vi "Search by MODEL.vi"(8 "error in (no error)":errorcluster, 10 "Device Info":T1, 11 "array of devices":T2) -> (0 "error out":errorcluster, 3 "Array":T1[](array[typedef]))   [LabVIEW 2016]
uses:
  Array Device Info.ctl
  Device Info.ctl
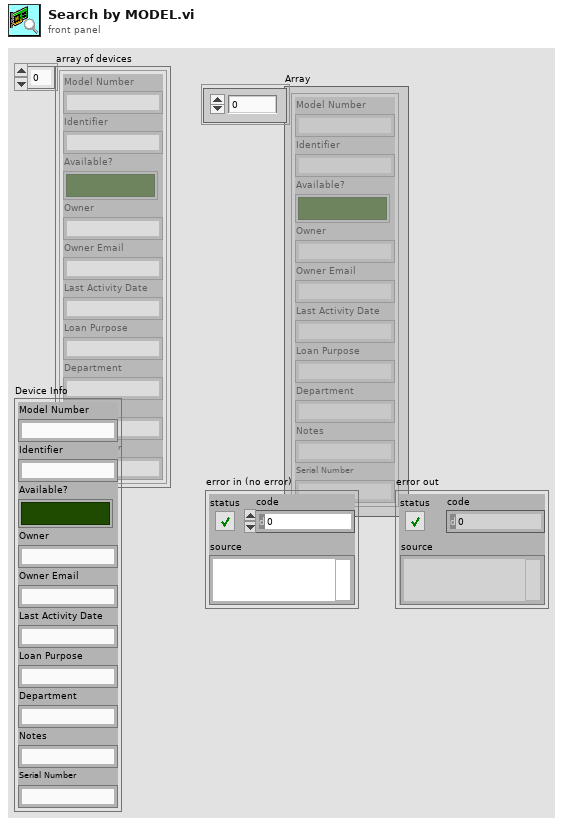
[diagram p1: front panel]
types:
  T1 = typedef "Device Info.ctl" = cluster{"Model Number":string, "Identifier":string, "Available?":bool, "Owner":string, "Owner Email":string, "Last Activity Date":string, "Loan Purpose":string, "Department":string, "Notes":string, "Serial Number":string}
  T2 = typedef "Array Device Info.ctl" = T1[]
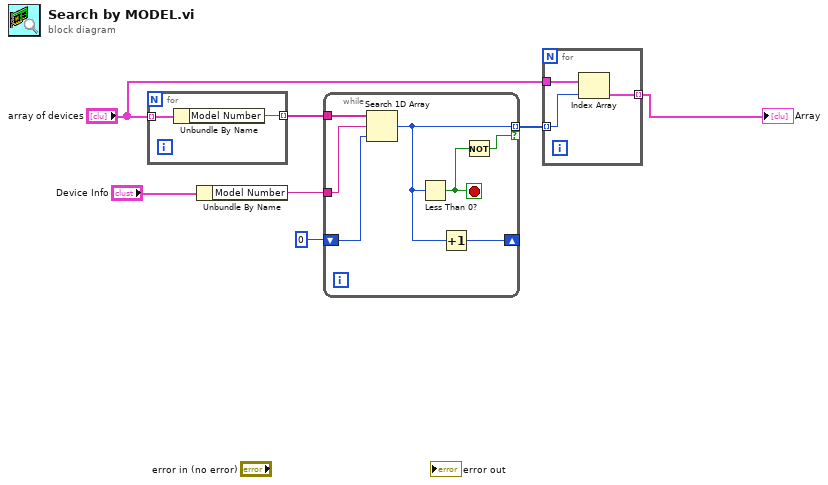
[diagram p0: block diagram]
diagram:
  n1 = for {
    tunnel: "array of devices" -> [w9] mode=indexing
    tunnel: [w8] -> w5 mode=indexing
    n2 = Unbundle By Name(w9) -> ("Model Number"=w8:string)
  }
  n3 = Unbundle By Name("Device Info") -> ("Model Number"=w3:string)
  n4 = while {
    tunnel: w5 -> [w16]
    tunnel: w3 -> [w15]
    tunnel: [w10] -> w4 mode=indexing if=w13
    shift-right: [w11] -> _
    shift-left: 0 -> [w12]
    stop <- w14 stop-if-true
    n5 = Search 1D Array(1D array=w16, element=w15, start index (0)=w12) -> (index of element=w10:i32)
    n6 = Less Than 0?(x=w10) -> (x < 0?=w14:bool)
    n7 = Increment(x=w10) -> (x+1=w11:i32)
    n8 = Not(x=w14) -> (.not. x?=w13:bool)
  }
  n9 = for {
    tunnel: w4 -> [w18] mode=indexing
    tunnel: "array of devices" -> [w19]
    tunnel: [w17] -> w6 mode=indexing
    n10 = Index Array(array=w19, index=w18) -> (element=w17:T1)
  }
  "Array" <- w6
